vi "Read Value.vi"(8 "error in (no error)":errorcluster, 11 "int32 in":refnum<class "sint32.lvclass">) -> (0 "error out":errorcluster, 2 "Value":i32, 3 "int32 out":refnum<class "sint32.lvclass">)   [LabVIEW 2020, in "Protobuf RAW.lvlib" / "sint32.lvclass"]
uses:
  sint32.lvclass
  sint32.lvclass/sint32.ctl
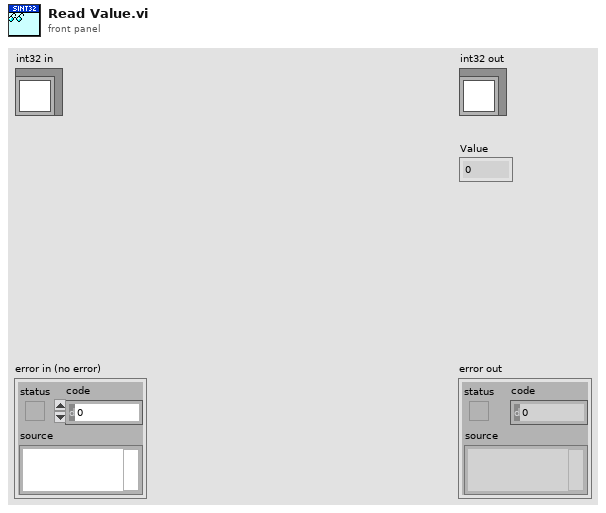
[diagram p1: front panel]
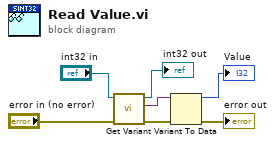
[diagram p0: block diagram]
diagram:
  n1 = call-dynamic "Get Variant.vi"("error in (no error)"="error in (no error)", "Proto Type Common in"="int32 in") -> ("error out"=w4:errorcluster, "Value"=w2:variant, "Proto Type Common out"=→"int32 out":refnum<class "sint32.lvclass">)  [unwired: 7 in]
  n2 = Variant To Data(error in=w4, Variant=w2) -> (data=→"Value":i32, error out=→"error out":errorcluster)  [unwired: 1 in]
